vi "Get Item PathName.vi"(8 "error in (no error)":errorcluster, 11 "Item Reference in":T1 format="%.0x") -> (0 "error out":errorcluster, 2 "PathName":string, 3 "Item Reference out":T1 format="%.0x", 4 "found":bool)   [LabVIEW 2013, in "Hierarchy Framework.lvlib" / "Item.lvclass"]
uses:
  Item.lvclass
  Ctls/Item Reference.ctl
  Generic/Generic.lvclass
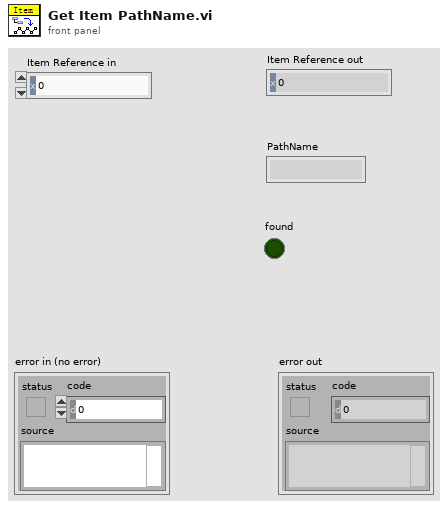
[diagram p1: front panel]
types:
  T1 = typedef "Hierarchy Framework.lvlib/Item.lvclass/Item Reference.ctl" = u64
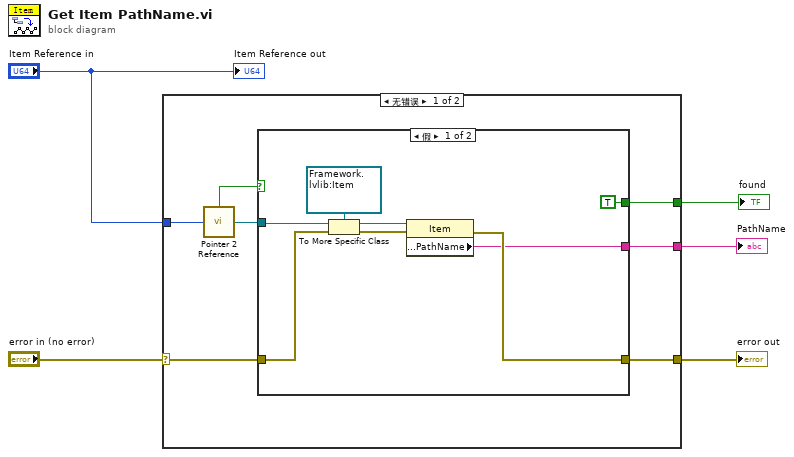
[diagram p0: block diagram]
diagram:
  n1 = case shown="无错误" "error in (no error)" {
    selector: "error in (no error)" -> [w11 w22]
    tunnel: "Item Reference in" -> [w10 _]
    tunnel: [w12 w22] -> w4
    tunnel: [w7 _] -> w2
    tunnel: [w6 _] -> w1
    frame No Error {
      n2 = call "Pointer 2 Reference.vi"("Pointer"=w10) -> ("Not A Refnum?"=w9:bool, "Generic Reference"=w8:refnum<data-value>)
      n3 = case shown="假" w9 {
        tunnel: w11 -> [w19 w21]
        tunnel: [w15 w21] -> w12
        tunnel: w8 -> [w20 _]
        tunnel: [w14 _] -> w7
        tunnel: [TRUE _] -> w6
        frame False {
          n4 = To More Specific Class(target class=refnum<data-value> refnum ("Item"), reference=w20, error in=w19) -> (specific class reference=w17:refnum<data-value>, error out=w16:errorcluster)
          n5 = property class="Item"(reference=w17, error in=w16) -> (error out=w15:errorcluster, "Accessors:PathName"=w14:string)  [unwired: 1 out]
        }
        frame True {
        }
      }
    }
    frame Error {
    }
  }
  "error out" <- w4
  "PathName" <- w2
  "found" <- w1
  "Item Reference out" <- "Item Reference in"
